vi "RM.renameDeviceReservationDB.vi"(8 "error in (no error)":errorcluster, 10 "Name":string, 11 "Device Ref in":T1 format="%.0x") -> (0 "error out":errorcluster, 2 "Request invalid?":bool, 3 "Device Ref out":T1=18446744073709551615 format="%.0x")   [LabVIEW 2016, in "FPGA Addon Shared.lvlib"]
uses:
  Shared/FPGA Addon Shared.lvlib
  <vilib>/NI Veristand/Custom Device API/Custom Device Item Ref.ctl
  <vilib>/NI VeriStand/Custom Device API/Custom Device API.lvlib
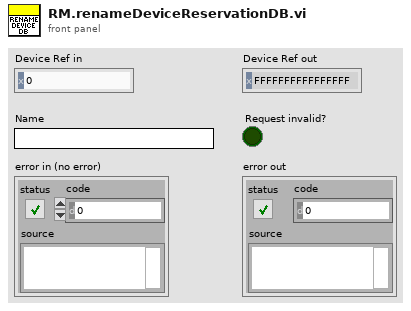
[diagram p1: front panel]
types:
  T1 = typedef "Custom Device API.lvlib/Custom Device Item Ref.ctl" = u64
  T2 = typedef "Custom Device API.lvlib/Custom Device Item Info.ctl" = cluster{"Name":string, "Is Channel":bool, "GUID":string, "Is Waveform":bool}
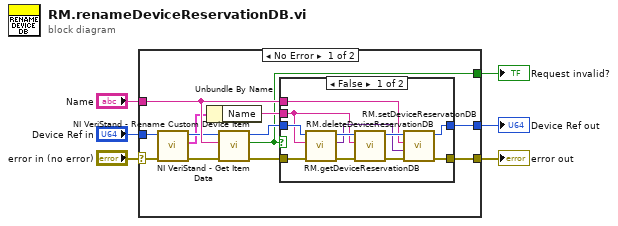
[diagram p0: block diagram]
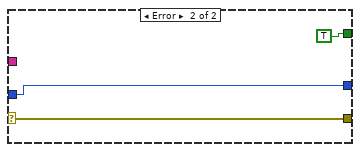
[diagram p3: hidden frame]
diagram:
  n1 = case shown="No Error" "error in (no error)" {
    selector: "error in (no error)" -> [w9 w33]
    tunnel: [w18 w34] -> w6
    tunnel: [w17 w33] -> w5
    tunnel: "Name" -> [w16 _]
    tunnel: [w10 TRUE ("Request invalid?")] -> w3
    tunnel: "Device Ref in" -> [w8 w34]
    frame No Error {
      n2 = call <vilib>:"NI VeriStand - Get Item Data.vi"("error in (no error)"=w9, "Item Ref in"=w8) -> ("error out"=w14:errorcluster, "Item Info"=w7:T2, "Item Ref out"=w13:T1)  [unwired: 7 out]
      n3 = Unbundle By Name(w7) -> ("Name"=w12:string)
      n4 = call <vilib>:"NI VeriStand - Rename Custom Device Item.vi"("error in (no error)"=w14, "New Name"=w16, "Item Ref in"=w13) -> ("error out"=w15:errorcluster, "Request invalid?"=w10:bool, "Item Ref out"=w11:T1)  [unwired: 1 in, 5 out]
      n5 = case shown="False" w10 {
        tunnel: w11 -> [w29 w31]
        tunnel: w12 -> [w19 _]
        tunnel: w15 -> [w25 w30]
        tunnel: w16 -> [w27 _]
        tunnel: [w21 w30] -> w17
        tunnel: [w20 w31] -> w18
        frame False {
          n6 = call "RM.getDeviceReservationDB.vi"("error in"=w25, "device name"=w19, "Item Ref in"=w29) -> ("error out"=w24:errorcluster, "reservation DB out"=w23:variant, "Item Ref out"=w26:T1)  [unwired: 5 in, 1 out]
          n7 = call "RM.deleteDeviceReservationDB.vi"("error in"=w24, "device name"=w19, "Item Ref in"=w26) -> ("error out"=w22:errorcluster, "Item Ref out"=w28:T1)  [unwired: 6 in, 1 out]
          n8 = call "RM.setDeviceReservationDB.vi"("error in"=w22, "reservation DB in"=w23, "device name"=w27, "Item Ref in"=w28) -> ("error out"=w21:errorcluster, "Item Ref out"=w20:T1)  [unwired: 5 in, 1 out]
        }
        frame True {
        }
      }
    }
    frame Error {
    }
  }
  "Device Ref out" <- w6
  "error out" <- w5
  "Request invalid?" <- w3
